vi "Console_writeLines.vi"(5 "New Lines":refnum<vi>, 7 "Console":refnum<vi>, 8 "error in (no error)":errorcluster, 9 "Console In":string, 10 "code":string, 11 "Python in":T1) -> (0 "error out":errorcluster, 1 "Console Out":string)   [LabVIEW 2022 SP3]
uses:
  PythonCtrl.ctl
  Processors.ctl
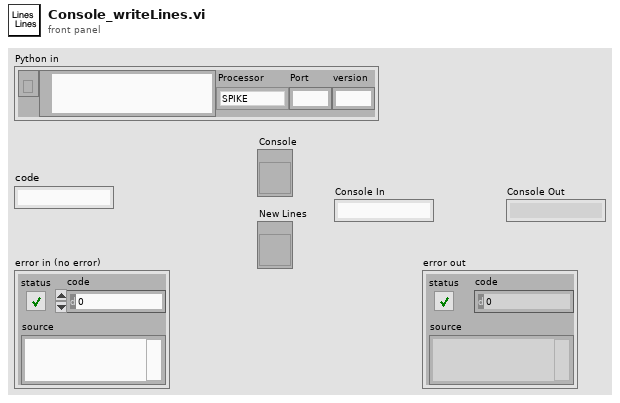
[diagram p1: front panel]
types:
  T1 = typedef "PythonCtrl.ctl" = cluster{"session":refnum<k35>, "PyPath":path, "Processor":T2, "Port":string, "version":string}
  T2 = typedef "Processors.ctl" = enum16{"SPIKE", "Pi", "Pi_ssh", "OpenMV", "Dunio"}
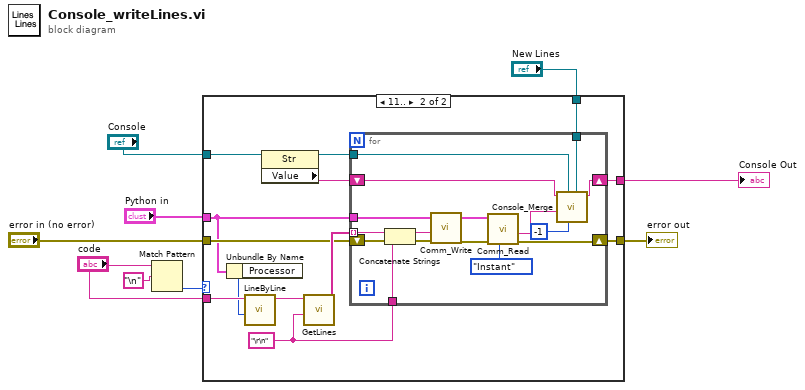
[diagram p0: block diagram]
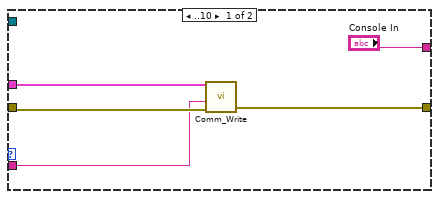
[diagram p2: hidden frame]
diagram:
  n1 = Match Pattern(string="code", regular expression="\n" ("delimiter")) -> (offset past match=w4:i32)  [unwired: 1 in, 3 out]
  n2 = case shown="11.." w4 {
    tunnel: "Python in" -> [w14 w22]
    tunnel: "code" -> [w11 w25]
    tunnel: [w13 w24] -> w8
    tunnel: "error in (no error)" -> [w12 w23]
    tunnel: "New Lines" -> [_ w19]
    tunnel: "Console" -> [_ w17]
    tunnel: ["Console In" w15] -> w1
    frame ..10 {
      n3 = call "Comm_Write.vi"("error in (no error)"=w12, "Text to write"=w11, "Python"=w14) -> ("error out"=w13:errorcluster)  [unwired: 7 in, 1 out]
    }
    frame 11.. {
      w20 = "\r\n" ("delimiter")
      n4 = Unbundle By Name(w22) -> ("Processor"=w21:T2)
      n5 = call "LineByLine.vi"("Processor"=w21, "Python Code"=w25) -> ("result string"=w26:string)  [unwired: 9 in]
      n6 = property class="Str"(reference=w17) -> (reference out=w16:refnum<vi>, "Value"=w18:string)  [unwired: 1 in, 1 out]
      n7 = call "GetLines.vi"("delimiter"=w20, "String"=w26) -> ("Array"=w27:string[])  [unwired: 9 in]
      n8 = for {
        tunnel: w22 -> [w35]
        shift-right: [w34] -> w24
        shift-left: w23 -> [w41]
        tunnel: w27 -> [w40] mode=indexing
        tunnel: w20 -> [w38]
        tunnel: w19 -> [w31]
        tunnel: w16 -> [w29]
        shift-right: [w30] -> w15
        shift-left: w18 -> [w28]
        n9 = Concatenate Strings(w40, w38) -> (w39:string)
        n10 = call "Comm_Write.vi"("error in (no error)"=w41, "Text to write"=w39, "Python"=w35) -> ("error out"=w36:errorcluster)  [unwired: 7 in, 1 out]
        n11 = call "Comm_Read.vi"("Task"=enum16{"Instant", "All", "AllFast", "Params"}."Instant", "error in (no error)"=w36, "Python"=w35) -> ("error out"=w34:errorcluster, "Text read"=w33:string)  [unwired: 7 in]
        n12 = call "Console_Merge.vi"("New Lines"=w31, "Buffer Size"=-1, "Console"=w29, "Text read"=w33, "Console In"=w28) -> ("Console Out"=w30:string)  [unwired: 6 in]
      }
    }
  }
  "error out" <- w8
  "Console Out" <- w1
